vi "GetModuleInfo.vi"(9 "Delta T":dbl, 11 "Module Positions In":T1[](array[typedef]) {"Angle"."SIN" format="%13.4f"; "Angle"."COS" format="%13.4f"; "Angle"."VALUE" format="%13.4f"}) -> (1 "Wheel States":T3[](array[typedef]) {"Angle"."SIN" format="%13.4f"; "Angle"."COS" format="%13.4f"; "Angle"."VALUE" format="%13.4f"}, 3 "Module Positions":T1[](array[typedef]) {"Angle"."SIN" format="%13.4f"; "Angle"."COS" format="%13.4f"; "Angle"."VALUE" format="%13.4f"})   [LabVIEW 2023]
uses:
  <vilib>/Rock Robotics/WPI/ThirdParty/JAS_Junk/TrajLib/TypeDef/SWERVE_DRIVE_MODULE_POSITION.ctl
  <vilib>/Rock Robotics/WPI/ThirdParty/JAS_Junk/TrajLib/TypeDef/ROTATION2D.ctl
  <vilib>/Rock Robotics/WPI/ThirdParty/JAS_Junk/TrajLib/TypeDef/SWERVE_DRIVE_MODULE_STATE.ctl
  <vilib>/Rock Robotics/WPI/ThirdParty/JAS_Junk/TrajLib/Trajectory_Library.lvlib
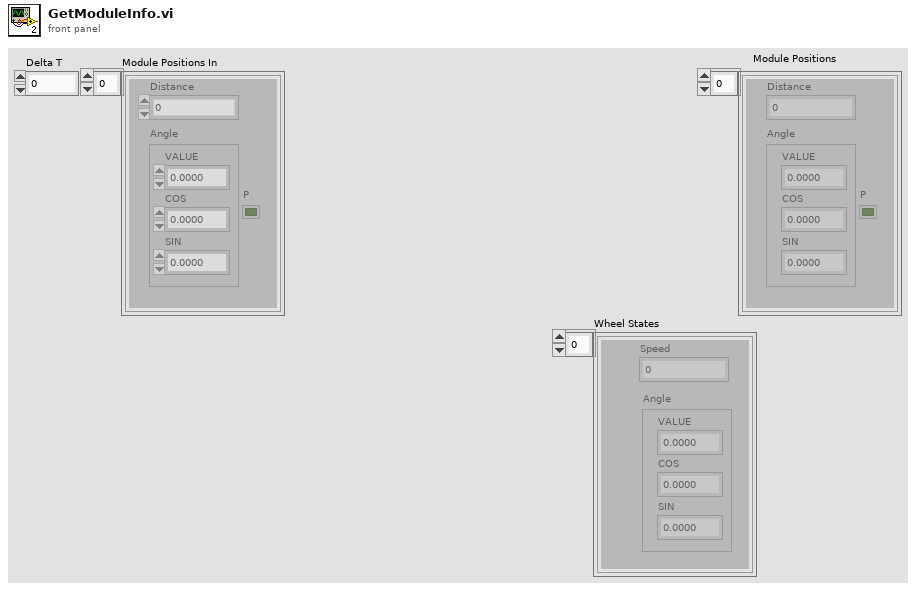
[diagram p1: front panel]
types:
  T1 = typedef "Trajectory_Library.lvlib/SWERVE_DRIVE_MODULE_POSITION.ctl" = cluster{"Distance":dbl, "Angle":T2, "P":bool}
  T2 = typedef "Trajectory_Library.lvlib/ROTATION2D.ctl" = cluster{"VALUE":dbl, "COS":dbl, "SIN":dbl}
  T3 = typedef "Trajectory_Library.lvlib/SWERVE_DRIVE_MODULE_STATE.ctl" = cluster{"Speed":dbl, "Angle":T2}
  T4 = typedef "WPI_MotorControlDeviceRef.ctl" = cluster{"DeviceStatus":errorcluster, "Type":T5, "PWM":cluster{"PWM Channel":T6, "DeadBand":T7}, "CAN":cluster{"Device Number":u8, "SetOutput VI Ref":variant, "GetOutput VI Ref":variant, "Enable VI Ref":variant, "Disable VI Ref":variant, "Data":variant}, "Invert":bool, "DIO PWM":cluster{"PWM \"Enable\" Channel":T6, "DIOChannel":T8, "PWM Rate":dbl}}
  T5 = typedef "WPI_MotorControlType.ctl" = enum16{"PWM", "CAN", "DIO PWM"}
  T6 = typedef "FPGA_DIOPWMChannel.ctl" = enum8{"PWM 0", "PWM 1", "PWM 2", "PWM 3", "PWM 4", "PWM 5", "PWM 6", "PWM 7", "PWM 8", "PWM 9", "PWM MXP 0", "PWM MXP 1", "PWM MXP 2", "PWM MXP 3", "PWM MXP 4", "PWM MXP 5", "PWM MXP 6", "PWM MXP 7", "PWM MXP 8", "PWM MXP 9", "Invalid"}
  T7 = typedef "WPI_PWMDeadband.ctl" = cluster{"Name":string, "maxPositivePwm":i32, "minPositivePwm":i32, "centerPwm":i32, "maxNegativePwm":i32, "minNegativePwm":i32, "angularRange":u16}
  T8 = typedef "FPGA_DIOChannel.ctl" = enum8{"DIO 0", "DIO 1", "DIO 2", "DIO 3", "DIO 4", "DIO 5", "DIO 6", "DIO 7", "DIO 8", "DIO 9", "DIO MXP 0", "DIO MXP 1", "DIO MXP 2", "DIO MXP 3", "DIO MXP 4", "DIO MXP 5", "DIO MXP 6", "DIO MXP 7", "DIO MXP 8", "DIO MXP 9", "DIO MXP 10", "DIO MXP 11", "DIO MXP 12", "DIO MXP 13", "DIO MXP 14", "DIO MXP 15", "SPI Port CS1", "SPI Port CS2", "SPI Port CS3", "SPI Port MISO", "SPI Port MOSI", "Invalid"}
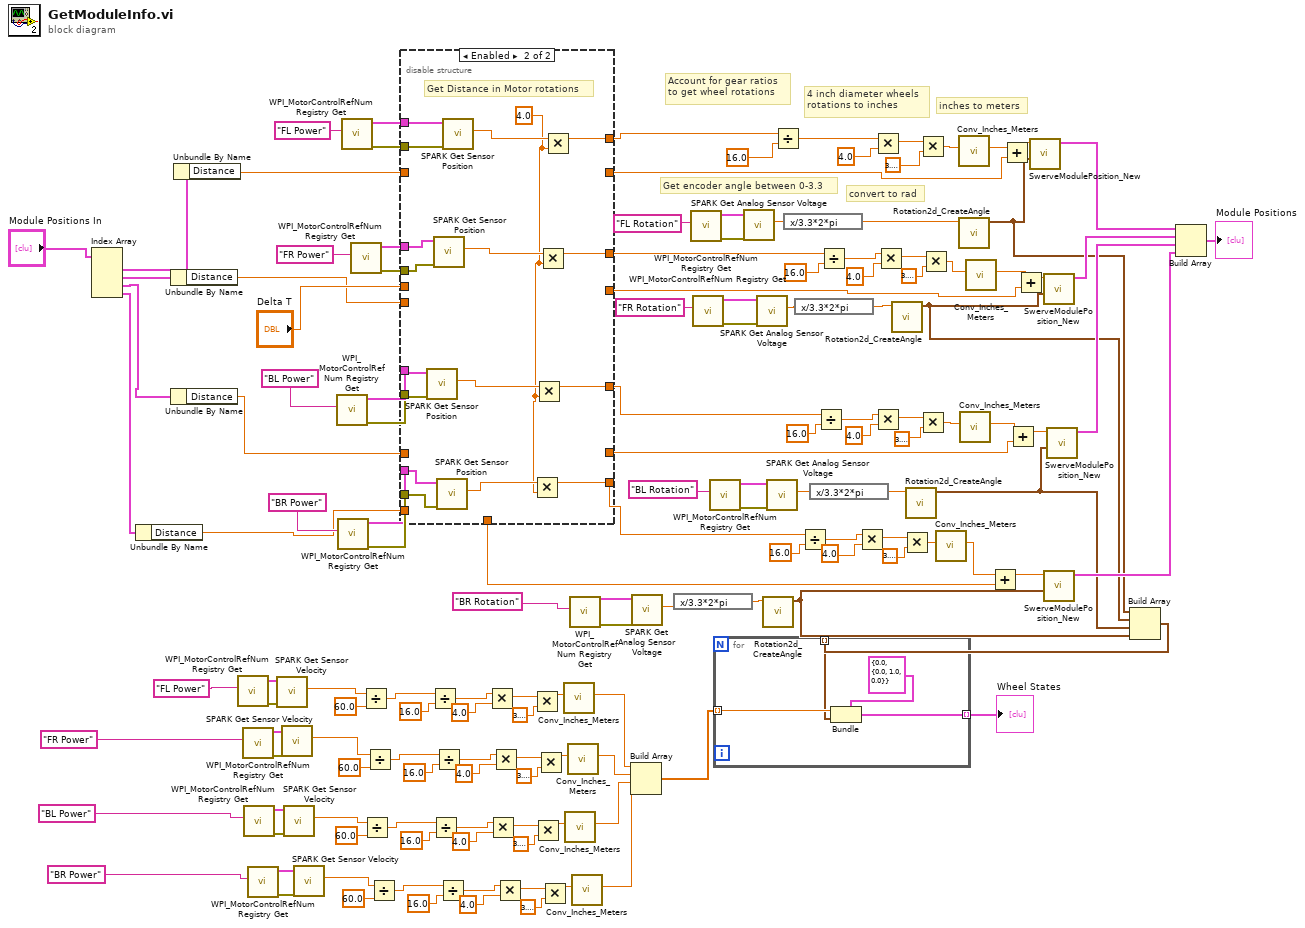
[diagram p0: block diagram]
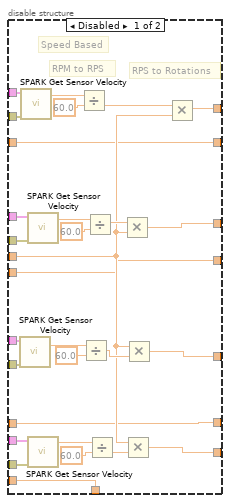
[diagram p2: hidden frame]
diagram:
  # "convert to rad"
  # "Get encoder angle between 0-3.3"
  # "inches to meters"
  # "4 inch diameter wheels\nrotations to inches"
  # "Account for gear ratios\nto get wheel rotations"
  n1 = Index Array(array="Module Positions In") -> (element #1=w16:T1, element #2=w14:T1, element #3=w13:T1, element #4=w15:T1)  [unwired: 4 in]
  n2 = Unbundle By Name(w15) -> ("Distance"=w1:dbl)
  n3 = Unbundle By Name(w14) -> ("Distance"=w8:dbl)
  n4 = Unbundle By Name(w13) -> ("Distance"=w10:dbl)
  n5 = Unbundle By Name(w16) -> ("Distance"=w4:dbl)
  n6 = call <vilib>:"WPI_MotorControlRefNum Registry Get.vi"("refnum name"="FL Power") -> ("error out"=w57:errorcluster, "MotorControlDevRef"=w56:T4)  [unwired: 9 in]
  n7 = call <vilib>:"WPI_MotorControlRefNum Registry Get.vi"("refnum name"="FR Power") -> ("error out"=w54:errorcluster, "MotorControlDevRef"=w55:T4)  [unwired: 9 in]
  n8 = call <vilib>:"WPI_MotorControlRefNum Registry Get.vi"("refnum name"="BL Power") -> ("error out"=w58:errorcluster, "MotorControlDevRef"=w59:T4)  [unwired: 9 in]
  n9 = call <vilib>:"WPI_MotorControlRefNum Registry Get.vi"("refnum name"="BR Power") -> ("error out"=w52:errorcluster, "MotorControlDevRef"=w53:T4)  [unwired: 9 in]
  n10 = call <vilib>:"SPARK Get Sensor Velocity.vi"("error in (no error)"=w57, "MotorControlDevRef in"=w56) -> ("Sensor Velocity"=w77:dbl)  [unwired: 6 in, 3 out]
  n11 = call <vilib>:"SPARK Get Sensor Velocity.vi"("error in (no error)"=w54, "MotorControlDevRef in"=w55) -> ("Sensor Velocity"=w78:dbl)  [unwired: 6 in, 3 out]
  n12 = call <vilib>:"SPARK Get Sensor Velocity.vi"("error in (no error)"=w58, "MotorControlDevRef in"=w59) -> ("Sensor Velocity"=w79:dbl)  [unwired: 6 in, 3 out]
  n13 = call <vilib>:"SPARK Get Sensor Velocity.vi"("error in (no error)"=w52, "MotorControlDevRef in"=w53) -> ("Sensor Velocity"=w62:dbl)  [unwired: 6 in, 3 out]
  n14 = call <vilib>:"WPI_MotorControlRefNum Registry Get.vi"("refnum name"="BL Power") -> ("error out"=w109:errorcluster, "MotorControlDevRef"=w110:T4)  [unwired: 9 in]
  n15 = call <vilib>:"WPI_MotorControlRefNum Registry Get.vi"("refnum name"="BR Power") -> ("error out"=w120:errorcluster, "MotorControlDevRef"=w119:T4)  [unwired: 9 in]
  n16 = call <vilib>:"WPI_MotorControlRefNum Registry Get.vi"("refnum name"="FL Power") -> ("error out"=w90:errorcluster, "MotorControlDevRef"=w91:T4)  [unwired: 9 in]
  n17 = call <vilib>:"WPI_MotorControlRefNum Registry Get.vi"("refnum name"="FR Power") -> ("error out"=w99:errorcluster, "MotorControlDevRef"=w100:T4)  [unwired: 9 in]
  n18 = Divide(x=w77, y=60.0) -> (x/y=w74:dbl)
  n19 = Divide(x=w79, y=60.0) -> (x/y=w66:dbl)
  n20 = Divide(x=w78, y=60.0) -> (x/y=w71:dbl)
  n21 = Divide(x=w62, y=60.0) -> (x/y=w63:dbl)
  n22 = disable-structure shown="Enabled" {
    disable-tunnel: [w152 w177] -> w122
    disable-tunnel: w120 -> [w172 w191]
    disable-tunnel: w119 -> [w171 w192]
    disable-tunnel: [w153 w178] -> w116
    disable-tunnel: w110 -> [w167 w189]
    disable-tunnel: w109 -> [w166 w190]
    disable-tunnel: [w154 w179] -> w103
    disable-tunnel: w100 -> [w162 w187]
    disable-tunnel: w99 -> [w161 w188]
    disable-tunnel: [w155 w180] -> w97
    disable-tunnel: w91 -> [w157 w185]
    disable-tunnel: w90 -> [w156 w186]
    disable-tunnel: "Delta T" -> [w151 _]
    disable-tunnel: w10 -> [w150 _]
    disable-tunnel: [w150 _] -> w9
    disable-tunnel: w8 -> [w149 _]
    disable-tunnel: [w149 _] -> w7
    disable-tunnel: [w148 _] -> w5
    disable-tunnel: w4 -> [w148 _]
    disable-tunnel: [w147 _] -> w2
    disable-tunnel: w1 -> [w147 _]
    frame Disabled {
      # "RPS to Rotations"
      # "RPM to RPS"
      # "Speed Based"
      n23 = call <vilib>:"SPARK Get Sensor Velocity.vi"("error in (no error)"=w166, "MotorControlDevRef in"=w167) -> ("Sensor Velocity"=w169:dbl)  [unwired: 6 in, 3 out]
      n24 = call <vilib>:"SPARK Get Sensor Velocity.vi"("error in (no error)"=w156, "MotorControlDevRef in"=w157) -> ("Sensor Velocity"=w159:dbl)  [unwired: 6 in, 3 out]
      n25 = call <vilib>:"SPARK Get Sensor Velocity.vi"("error in (no error)"=w161, "MotorControlDevRef in"=w162) -> ("Sensor Velocity"=w164:dbl)  [unwired: 6 in, 3 out]
      n26 = call <vilib>:"SPARK Get Sensor Velocity.vi"("error in (no error)"=w172, "MotorControlDevRef in"=w171) -> ("Sensor Velocity"=w174:dbl)  [unwired: 6 in, 3 out]
      n27 = Divide(x=w159, y=60.0) -> (x/y=w160:dbl)
      n28 = Divide(x=w169, y=60.0) -> (x/y=w170:dbl)
      n29 = Divide(x=w164, y=60.0) -> (x/y=w163:dbl)
      n30 = Divide(x=w174, y=60.0) -> (x/y=w173:dbl)
      n31 = Multiply(x=w163, y=w151) -> (x*y=w154:dbl)
      n32 = Multiply(x=w151, y=w173) -> (x*y=w152:dbl)
      n33 = Multiply(x=w151, y=w170) -> (x*y=w153:dbl)
      n34 = Multiply(x=w160, y=w151) -> (x*y=w155:dbl)
    }
    frame Enabled {
      w176 = 4.0 ("y")
      # "Get Distance in Motor rotations"
      n35 = call <vilib>:"SPARK Get Sensor Position.vi"("error in (no error)"=w190, "MotorControlDevRef in"=w189) -> ("Sensor Position"=w182:dbl)  [unwired: 6 in, 3 out]
      n36 = call <vilib>:"SPARK Get Sensor Position.vi"("error in (no error)"=w188, "MotorControlDevRef in"=w187) -> ("Sensor Position"=w183:dbl)  [unwired: 6 in, 3 out]
      n37 = call <vilib>:"SPARK Get Sensor Position.vi"("error in (no error)"=w191, "MotorControlDevRef in"=w192) -> ("Sensor Position"=w181:dbl)  [unwired: 6 in, 3 out]
      n38 = call <vilib>:"SPARK Get Sensor Position.vi"("error in (no error)"=w186, "MotorControlDevRef in"=w185) -> ("Sensor Position"=w184:dbl)  [unwired: 6 in, 3 out]
      n39 = Multiply(x=w181, y=w176) -> (x*y=w177:dbl)
      n40 = Multiply(x=w182, y=w176) -> (x*y=w178:dbl)
      n41 = Multiply(x=w183, y=w176) -> (x*y=w179:dbl)
      n42 = Multiply(x=w184, y=w176) -> (x*y=w180:dbl)
    }
  }
  n43 = Divide(x=w74, y=16.0) -> (x/y=w75:dbl)
  n44 = Divide(x=w66, y=16.0) -> (x/y=w67:dbl)
  n45 = Divide(x=w71, y=16.0) -> (x/y=w70:dbl)
  n46 = Divide(x=w63, y=16.0) -> (x/y=w61:dbl)
  n47 = Multiply(x=w75, y=4.0) -> (x*y=w76:dbl)
  n48 = Multiply(x=w67, y=4.0) -> (x*y=w68:dbl)
  n49 = Multiply(x=w70, y=4.0) -> (x*y=w69:dbl)
  n50 = Multiply(x=w61, y=4.0) -> (x*y=w60:dbl)
  n51 = Multiply(x=w76, y=3.141592653589793) -> (x*y=w73:dbl)
  n52 = Multiply(x=w68, y=3.141592653589793) -> (x*y=w65:dbl)
  n53 = Multiply(x=w69, y=3.141592653589793) -> (x*y=w72:dbl)
  n54 = Multiply(x=w60, y=3.141592653589793) -> (x*y=w64:dbl)
  n55 = call <vilib>:"Conv_Inches_Meters.vi"("INCH"=w73) -> ("Meters"=w31:dbl)  [unwired: 10 in]
  n56 = call <vilib>:"Conv_Inches_Meters.vi"("INCH"=w65) -> ("Meters"=w28:dbl)  [unwired: 10 in]
  n57 = call <vilib>:"Conv_Inches_Meters.vi"("INCH"=w72) -> ("Meters"=w30:dbl)  [unwired: 10 in]
  n58 = call <vilib>:"WPI_MotorControlRefNum Registry Get.vi"("refnum name"="BR Rotation") -> ("error out"=w85:errorcluster, "MotorControlDevRef"=w135:T4)  [unwired: 9 in]
  n59 = call <vilib>:"Conv_Inches_Meters.vi"("INCH"=w64) -> ("Meters"=w29:dbl)  [unwired: 10 in]
  n60 = Build Array(w31, w30, w28, w29) -> (w27:dbl[])
  n61 = call <vilib>:"SPARK Get Analog Sensor Voltage.vi"("error in (no error)"=w85, "MotorControlDevRef in"=w135) -> ("Analog Sensor Voltage"=w133:dbl)  [unwired: 6 in, 3 out]
  n62 = expression code="x/3.3*2*pi"(w133) -> (w26:dbl)
  n63 = call <vilib>:"WPI_MotorControlRefNum Registry Get.vi"("refnum name"="FL Rotation") -> ("error out"=w82:errorcluster, "MotorControlDevRef"=w138:T4)  [unwired: 9 in]
  n64 = call <vilib>:"WPI_MotorControlRefNum Registry Get.vi"("refnum name"="FR Rotation") -> ("error out"=w83:errorcluster, "MotorControlDevRef"=w137:T4)  [unwired: 9 in]
  n65 = call <vilib>:"WPI_MotorControlRefNum Registry Get.vi"("refnum name"="BL Rotation") -> ("error out"=w84:errorcluster, "MotorControlDevRef"=w136:T4)  [unwired: 9 in]
  n66 = call <vilib>:"SPARK Get Analog Sensor Voltage.vi"("error in (no error)"=w82, "MotorControlDevRef in"=w138) -> ("Analog Sensor Voltage"=w131:dbl)  [unwired: 6 in, 3 out]
  n67 = call <vilib>:"SPARK Get Analog Sensor Voltage.vi"("error in (no error)"=w83, "MotorControlDevRef in"=w137) -> ("Analog Sensor Voltage"=w134:dbl)  [unwired: 6 in, 3 out]
  n68 = call <vilib>:"Rotation2d_CreateAngle.vi"("Angle"=w26) -> ("ROTATION"=w25:T2)  [unwired: 10 in]
  n69 = call <vilib>:"SPARK Get Analog Sensor Voltage.vi"("error in (no error)"=w84, "MotorControlDevRef in"=w136) -> ("Analog Sensor Voltage"=w132:dbl)  [unwired: 6 in, 3 out]
  n70 = Divide(x=w97, y=16.0) -> (x/y=w96:dbl)
  n71 = expression code="x/3.3*2*pi"(w131) -> (w130:dbl)
  n72 = expression code="x/3.3*2*pi"(w134) -> (w129:dbl)
  n73 = Divide(x=w122, y=16.0) -> (x/y=w123:dbl)
  n74 = expression code="x/3.3*2*pi"(w132) -> (w128:dbl)
  n75 = Divide(x=w116, y=16.0) -> (x/y=w115:dbl)
  n76 = Divide(x=w103, y=16.0) -> (x/y=w104:dbl)
  n77 = Multiply(x=w123, y=4.0) -> (x*y=w125:dbl)
  n78 = Multiply(x=w96, y=4.0) -> (x*y=w94:dbl)
  n79 = Multiply(x=w115, y=4.0) -> (x*y=w113:dbl)
  n80 = Multiply(x=w104, y=4.0) -> (x*y=w106:dbl)
  n81 = call <vilib>:"Rotation2d_CreateAngle.vi"("Angle"=w129) -> ("ROTATION"=w23:T2)  [unwired: 10 in]
  n82 = Multiply(x=w125, y=3.141592653589793) -> (x*y=w127:dbl)
  n83 = call <vilib>:"Rotation2d_CreateAngle.vi"("Angle"=w128) -> ("ROTATION"=w24:T2)  [unwired: 10 in]
  n84 = Multiply(x=w94, y=3.141592653589793) -> (x*y=w93:dbl)
  n85 = Multiply(x=w113, y=3.141592653589793) -> (x*y=w111:dbl)
  n86 = Multiply(x=w106, y=3.141592653589793) -> (x*y=w107:dbl)
  n87 = call <vilib>:"Conv_Inches_Meters.vi"("INCH"=w127) -> ("Meters"=w118:dbl)  [unwired: 10 in]
  n88 = call <vilib>:"Conv_Inches_Meters.vi"("INCH"=w93) -> ("Meters"=w92:dbl)  [unwired: 10 in]
  n89 = call <vilib>:"Rotation2d_CreateAngle.vi"("Angle"=w130) -> ("ROTATION"=w22:T2)  [unwired: 10 in]
  n90 = call <vilib>:"Conv_Inches_Meters.vi"("INCH"=w111) -> ("Meters"=w108:dbl)  [unwired: 10 in]
  n91 = call <vilib>:"Conv_Inches_Meters.vi"("INCH"=w107) -> ("Meters"=w101:dbl)  [unwired: 10 in]
  n92 = Add(x=w118, y=w2) -> (x+y=w3:dbl)
  n93 = Add(x=w92, y=w5) -> (x+y=w6:dbl)
  n94 = Add(x=w108, y=w9) -> (x+y=w11:dbl)
  n95 = Add(x=w101, y=w7) -> (x+y=w12:dbl)
  n96 = call <vilib>:"SwerveModulePosition_New.vi"("ROTATION"=w22, "Distance"=w6) -> ("SWERVE_DRIVE_MODULE_POSITION"=w89:T1)  [unwired: 9 in]
  n97 = call <vilib>:"SwerveModulePosition_New.vi"("ROTATION"=w23, "Distance"=w12) -> ("SWERVE_DRIVE_MODULE_POSITION"=w88:T1)  [unwired: 9 in]
  n98 = call <vilib>:"SwerveModulePosition_New.vi"("ROTATION"=w25, "Distance"=w3) -> ("SWERVE_DRIVE_MODULE_POSITION"=w86:T1)  [unwired: 9 in]
  n99 = call <vilib>:"SwerveModulePosition_New.vi"("ROTATION"=w24, "Distance"=w11) -> ("SWERVE_DRIVE_MODULE_POSITION"=w87:T1)  [unwired: 9 in]
  n100 = Build Array(w22, w23, w24, w25) -> (w21:T2[])
  n101 = for {
    tunnel: w27 -> [w196] mode=indexing
    tunnel: w21 -> [w195] mode=indexing
    tunnel: [w194] -> w18 mode=indexing
    n102 = Bundle(cluster=T3 {"Speed"=0.0, "Angle"={"VALUE"=0.0, "COS"=1.0, "SIN"=0.0}} ("SWERVE_DRIVE_MODULE_STATE"), "Speed"=w196, "Angle"=w195) -> (w194:T3)
  }
  "Wheel States" <- w18
  n103 = Build Array(w89, w88, w87, w86) -> (→"Module Positions":T1[])
